vi "Pulping_Process (SubVI).vi"(10 "Array in":string[](array[string]), 11 "Digital in":refnum<vi>) -> (1 "Array out":string[](array[string]), 2 "Boolean":bool, 3 "empty?":bool)   [LabVIEW 2019]
uses:
  b3f8d96a-64a2-407c-a638-ce800749bb10.vi
  <vilib>/numeric/Random Number (Range) DBL.vi
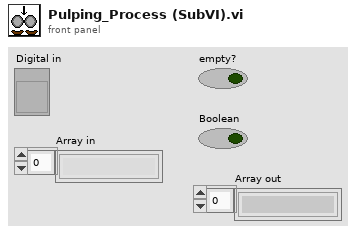
[diagram p1: front panel]
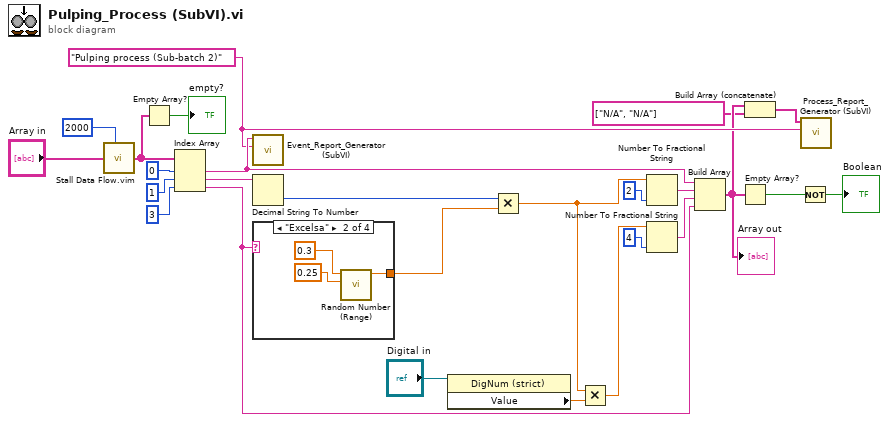
[diagram p0: block diagram]
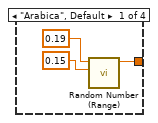
[diagram p2: hidden frame]
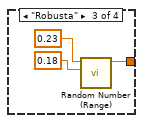
[diagram p3: hidden frame]
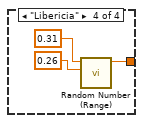
[diagram p4: hidden frame]
diagram:
  w4 = "Pulping process (Sub-batch 2)" ("Process Name")
  n1 = call "Stall Data Flow.vim"("value in"="Array in", "milliseconds to wait"=u32 2000) -> ("value out"=w24:string[])  [unwired: 1 out]
  n2 = Empty Array?(array=w24) -> (empty?=→"empty?":bool)
  n3 = Index Array(array=w24, index #1=0 ("index"), index #2=1 ("index"), index #3=3 ("index")) -> (element #1=w5:string, element #2=w9:string, element #3=w19:string)
  n4 = call "Event_Report_Generator (SubVI).vi"("Process Name"=w4, "Booking ID"=w5) -> ()  [unwired: 10 in]
  n5 = Decimal String To Number(string=w9) -> (number=w11:i32)  [unwired: 2 in, 1 out]
  n6 = case shown="\"Excelsa\"" w19 {
    tunnel: [w27 w30 w33 w36] -> w10
    frame "Arabica", Default {
      n7 = call-poly <vilib>:"Random Number (Range).vi"("lower bound (0)"=0.15, "upper bound (100)"=0.19) -> ("number"=w27:dbl)  [unwired: 9 in]
    }
    frame "Excelsa" {
      n8 = call-poly <vilib>:"Random Number (Range).vi"("lower bound (0)"=0.25, "upper bound (100)"=0.3) -> ("number"=w30:dbl)  [unwired: 9 in]
    }
    frame "Robusta" {
      n9 = call-poly <vilib>:"Random Number (Range).vi"("lower bound (0)"=0.18, "upper bound (100)"=0.23) -> ("number"=w33:dbl)  [unwired: 9 in]
    }
    frame "Libericia" {
      n10 = call-poly <vilib>:"Random Number (Range).vi"("lower bound (0)"=0.26, "upper bound (100)"=0.31) -> ("number"=w36:dbl)  [unwired: 9 in]
    }
  }
  n11 = property class="DigNum (strict)"(reference="Digital in") -> ("Value"=w20:dbl)  [unwired: 1 in, 2 out]
  n12 = Multiply(x=w11, y=w10) -> (x*y=w17:dbl)
  n13 = Multiply(x=w17, y=w20) -> (x*y=w16:dbl)
  n14 = Number To Fractional String(number=w17, precision (6)=i16 2) -> (F-format string=w13:string)  [unwired: 2 in]
  n15 = Number To Fractional String(number=w16, precision (6)=i16 4) -> (F-format string=w18:string)  [unwired: 2 in]
  n16 = Build Array(w5, w13, w18, w19) -> (w3:string[])
  "Array out" <- w3
  n17 = Empty Array?(array=w3) -> (empty?=w21:bool)
  n18 = Build Array (concatenate)(w3, string[] ["N/A", "N/A"] ("array")) -> (w2:string[])
  n19 = Not(x=w21) -> (.not. x?=→"Boolean":bool)
  n20 = call "Process_Report_Generator (SubVI).vi"("Process Name"=w4, "Process Information"=w2) -> ()  [unwired: 10 in]
